vi "Perform Action DataSocket Reply.vi"(6 "DataSocket Reply URL":string, 8 "error in":errorcluster, 9 "Input":variant, 10 "Task.Point Ident":string, 11 "MSS Target Actor in":refnum<class "MSS Target Actor.lvclass">) -> (0 "error out":errorcluster, 3 "MSS Target Actor out":refnum<class "MSS Target Actor.lvclass">)   [LabVIEW 2024, in "MSS Target Actor.lvlib" / "MSS Target Actor.lvclass"]
uses:
  MSS Target Actor.lvclass
  MSS Target Actor.lvclass/MSS Target Actor.ctl
  MSS/MSS.lvclass
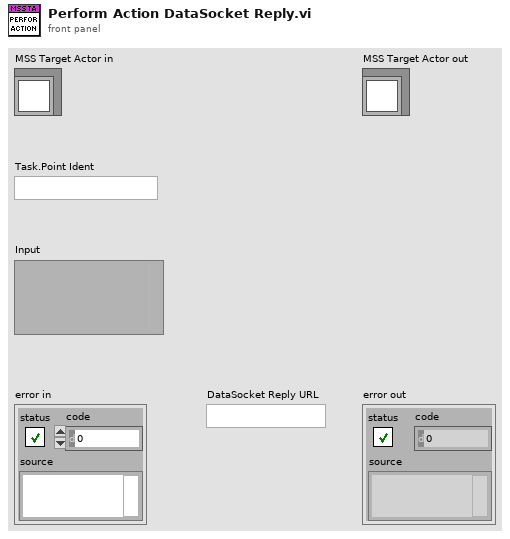
[diagram p1: front panel]
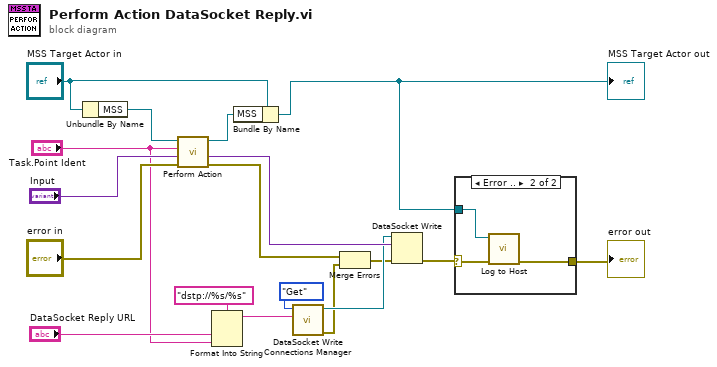
[diagram p0: block diagram]
diagram:
  n1 = Unbundle By Name("MSS Target Actor in") -> ("MSS"=w18:refnum<class "MSS.lvclass">)
  n2 = call "Perform Action.vi"("error in"="error in", "Input"="Input", "Point Ident"="Task.Point Ident", "MSS in"=w18) -> ("error out"=w13:errorcluster, "Output"=w12:variant, "MSS out"=w14:refnum<class "MSS.lvclass">)  [unwired: 4 in, 1 out]
  n3 = Format Into String(format string="dstp://%s/%s", "DataSocket Reply URL", "Task.Point Ident") -> (resulting string=w6:string)  [unwired: 2 in, 1 out]
  n4 = Bundle By Name(cluster="MSS Target Actor in", "MSS"=w14) -> (w3:refnum<class "MSS Target Actor.lvclass">)
  "MSS Target Actor out" <- w3
  n5 = call "DataSocket Write Connections Manager.vi"("URL"=w6, "Action"=enum16{"Get", "Close", "Close All"}."Get") -> ("error out"=w1:errorcluster, "connection id"=w10:refnum<k13>)  [unwired: 8 in]
  n6 = Merge Errors(w13, w1) -> (w2:errorcluster)
  n7 = DataSocket Write(8:w2, 10:w12, 11:w10) -> (0:w5:errorcluster)  [unwired: 1 in, 2 out]
  n8 = case shown="Error .." w5 {
    selector: w5 -> [w19 w22]
    tunnel: [w19 w21] -> w4
    tunnel: w3 -> [_ w20]
    frame No Error {
    }
    frame Error {
      n9 = call "Log to Host.vi"("error in"=w22, "MSS Target Actor in"=w20) -> ("error out"=w21:errorcluster)  [unwired: 8 in, 1 out]
    }
  }
  "error out" <- w4
